vi "HK Channel Get Table of Channels.vi"(8 "error in (no error)":errorcluster, 11 "HK Channel in":refnum<class "HK Table.lvclass">) -> (0 "error out":errorcluster, 1 "Header":string[](array[string]), 2 "Table":string[][](array[string]), 3 "HK Channel out":refnum<class "HK Table.lvclass">, 4 "Ch Names":string[](array[string]))   [LabVIEW 2024, in "HK Table.lvclass"]
uses:
  HK Table.lvclass
  HK Table.lvclass/HK Table.ctl
  HK Item/HK Item.lvclass/HK Item.ctl
  HK Alarms/HK Alarms.lvclass/HK Alarms.ctl
  HK Alarms/HK Alarms.lvclass
  HK Item/HK Item.lvclass
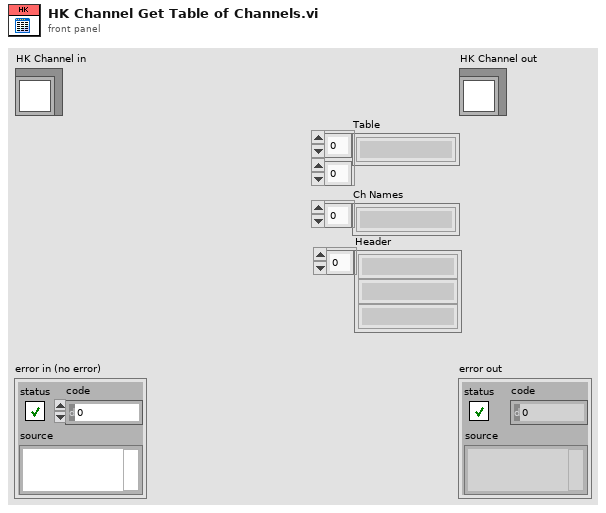
[diagram p1: front panel]
types:
  T1 = typedef "HK Item.lvclass/HK Channel Units and Setup.ctl" = cluster{"Unit Type":string, "Units":string, "Configuration":string, "Digits":i32, "Data Type":T2, "Exponential?":bool, "Source":string}
  T2 = typedef "HK Item.lvclass/HK Channel enum Data Type.ctl" = enum16{"Floating Point", "Integer", "Enum", "String", "Waveform", "File"}
  T3 = typedef "HK Item.lvclass/HK Channel Settings Physical.ctl" = cluster{"Type":string, "Device":string, "Module":string, "Channel":i32}
  T4 = typedef "HK Item.lvclass/HK Channel Settings Limits.ctl" = cluster{"Low Red":dbl, "Low Yellow":dbl, "Hi Yellow":dbl, "Hi Red":dbl}
  T5 = typedef "HK Item.lvclass/HK Channel Settings Scaling.ctl" = cluster{"Scaling Type":T6, "Parameters":dbl[]}
  T6 = typedef "HK Item.lvclass/HK Channel enum Scaling Type.ctl" = enum16{"None", "Polynomial"}
  T7 = typedef "HK Item.lvclass/HK Channel Settings Alarms.ctl" = cluster{"Enabled":bool, "Deadband":i32, "Action":T8}
  T8 = typedef "HK Item.lvclass/HK Alarm enum Action.ctl" = enum16{"Light", "Message", "Safe"}
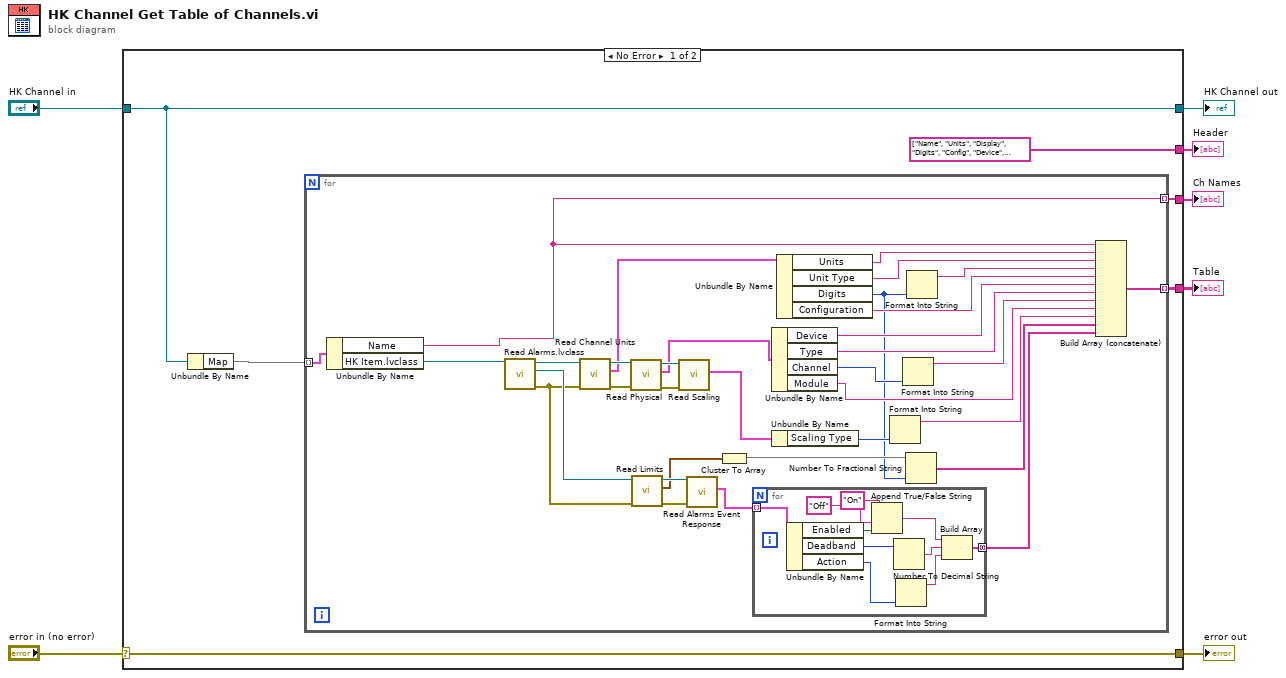
[diagram p0: block diagram]
diagram:
  n1 = case shown="No Error" "error in (no error)" {
    selector: "error in (no error)" -> [w13 w58]
    tunnel: [w13 w58] -> w6
    tunnel: [w11 w57] -> w4
    tunnel: "HK Channel in" -> [w11 w57]
    tunnel: [w10 _] -> w3
    tunnel: [w9 _] -> w2
    tunnel: [string[] ["Name", "Units", "Display", "Digits", "Config", "Device", "Device Type", "Channel", "Module", "Scaling Type", "Low Red", "Low Yellow", "High Yellow", "High Red", "Low Red Enable", "Low Red Deadband", "Low Red Action", "Low Yellow Enable", "Low Yellow Deadband", "Low Yellow Action", "High Yellow Enable", "High Yellow Deadband", "High Yellow Action", "High Red Enable", "High Red Deadband", "High Red Action"] _] -> w1
    frame No Error {
      n2 = Unbundle By Name(w11) -> ("Map"=w12:map{string, refnum<class "HK Item.lvclass">})
      n3 = for {
        tunnel: w12 -> [w46] mode=indexing
        tunnel: [w16] -> w10 mode=indexing
        tunnel: [w14] -> w9 mode=indexing
        n4 = Unbundle By Name(w46) -> ("Name"=w14:string, "HK Item.lvclass"=w15:refnum<class "HK Item.lvclass">)
        n5 = call "Read Alarms.lvclass.vi"("HK Item in"=w15) -> ("error out"=w38:errorcluster, "Alarms.lvclass"=w41:refnum<class "HK Alarms.lvclass">, "HK Item out"=w43:refnum<class "HK Item.lvclass">)  [unwired: 8 in]
        n6 = call "Read Channel Units.vi"("error in (no error)"=w38, "HK Item in"=w43) -> ("error out"=w40:errorcluster, "Channel Setup"=w36:T1, "HK Item out"=w45:refnum<class "HK Item.lvclass">)  [unwired: 7 in]
        n7 = call "Read Physical.vi"("error in (no error)"=w40, "HK Item in"=w45) -> ("error out"=w39:errorcluster, "Physical"=w31:T3, "HK Item out"=w44:refnum<class "HK Item.lvclass">)  [unwired: 7 in]
        n8 = call "Read Limits.vi"("error in (no error)"=w38, "Alarms in"=w41) -> ("error out"=w37:errorcluster, "Limits"=w22:T4, "Alarms out"=w42:refnum<class "HK Alarms.lvclass">)  [unwired: 7 in]
        n9 = call "Read Scaling.vi"("error in (no error)"=w39, "HK Item in"=w44) -> ("Scaling"=w25:T5)  [unwired: 7 in, 2 out]
        n10 = call "Read Alarms Event Response.vi"("error in (no error)"=w37, "Alarms in"=w42) -> ("Alarms"=w18:T7[])  [unwired: 7 in, 2 out]
        n11 = Cluster To Array(cluster=w22) -> (array=w21:dbl[])
        n12 = for {
          tunnel: w18 -> [w56] mode=indexing
          tunnel: [w47] -> w17 mode=concatenating
          n13 = Unbundle By Name(w56) -> ("Enabled"=w55:bool, "Deadband"=w52:i32, "Action"=w51:T8)
          n14 = Append True/False String(1:w55, 2:"Off" ("true string"), 3:"On" ("true string")) -> (0:w48:string)  [unwired: 1 in]
          n15 = Number To Decimal String(number=w52) -> (decimal integer string=w49:string)  [unwired: 1 in]
          n16 = Format Into String(w51) -> (resulting string=w50:string)  [unwired: 3 in, 1 out]
          n17 = Build Array(w48, w49, w50) -> (w47:string[])
        }
        n18 = Unbundle By Name(w31) -> ("Device"=w30:string, "Type"=w29:string, "Channel"=w28:i32, "Module"=w26:string)
        n19 = Unbundle By Name(w25) -> ("Scaling Type"=w24:T6)
        n20 = Unbundle By Name(w36) -> ("Units"=w35:string, "Unit Type"=w34:string, "Digits"=w20:i32, "Configuration"=w32:string)
        n21 = Format Into String(w24) -> (resulting string=w23:string)  [unwired: 3 in, 1 out]
        n22 = Format Into String(w28) -> (resulting string=w27:string)  [unwired: 3 in, 1 out]
        n23 = Number To Fractional String(number=w21, precision (6)=w20) -> (F-format string=w19:string[])  [unwired: 2 in]
        n24 = Format Into String(w20) -> (resulting string=w33:string)  [unwired: 3 in, 1 out]
        n25 = Build Array (concatenate)(w14, w35, w34, w33, w32, w30, w29, w27, w26, w23, w19, w17) -> (w16:string[])
      }
    }
    frame Error {
    }
  }
  "error out" <- w6
  "HK Channel out" <- w4
  "Table" <- w3
  "Ch Names" <- w2
  "Header" <- w1
